vi "Check Save to Disk Signal and Create or Close File.vi"(8 "error in (no error)":errorcluster, 11 "Save to Disk?":bool) -> (0 "error out":errorcluster)   [LabVIEW 2013]
doc: "Checks the Save to Disk? signal for a rising edge and then creates a file. If falling edge, then close the file. Otherwise do nothing."
uses:
  File IO/Save Image Module Enum.ctl
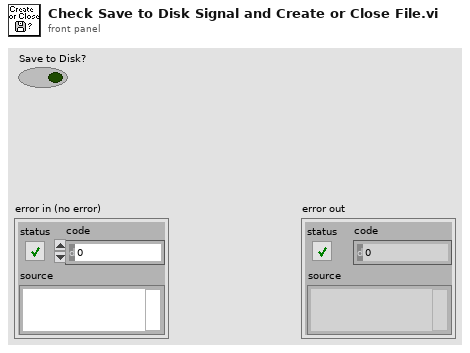
[diagram p1: front panel]
types:
  T1 = typedef "Save Image Module Enum.ctl" = enum16{"Create File", "Write to File", "Close File"}
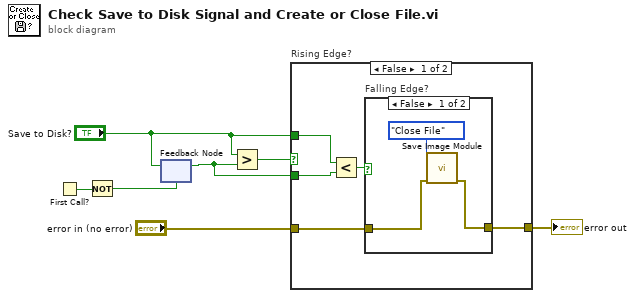
[diagram p0: block diagram]
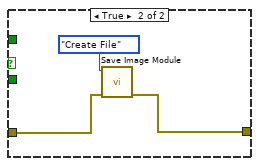
[diagram p3: hidden frame]
diagram:
  n1 = First Call?() -> (First Call?: T/F=w7:bool)
  n2 = Not(x=w7) -> (.not. x?=w6:bool)
  n3 = feedback #1(w6) -> (w1:bool)
  n4 = feedback-in #1("Save to Disk?") -> ()
  n5 = Greater?(x="Save to Disk?", y=w1) -> (0:w5:bool)
  n6 = case "Rising Edge?" shown="False" w5 {
    tunnel: "error in (no error)" -> [w9 w18]
    tunnel: [w8 w17] -> w3
    tunnel: "Save to Disk?" -> [w12 _]
    tunnel: w1 -> [w11 _]
    frame False {
      n7 = Less?(x=w12, y=w11) -> (x < y?=w10:bool)
      n8 = case "Falling Edge?" shown="False" w10 {
        tunnel: w9 -> [w14 w16]
        tunnel: [w13 w16] -> w8
        frame False {
          n9 = call "Save Image Module.vi"("error in"=w14, "Mode"=Save_Image_Module_Enum."Close File") -> ("error out"=w13:errorcluster)  [unwired: 9 in]
        }
        frame True {
        }
      }
    }
    frame True {
      n10 = call "Save Image Module.vi"("error in"=w18, "Mode"=Save_Image_Module_Enum."Create File") -> ("error out"=w17:errorcluster)  [unwired: 9 in]
    }
  }
  "error out" <- w3
